vi "Configure Spectral (Other).vi"(0 "VISA resource name":refnum<visa-resource-name>, 1 "Frequency Span (100kHz)":dbl=100000.0, 2 "Resolution BW (400Hz)":dbl=400000.0, 3 "Gate Position (0s)":dbl, 5 "Channel (4:Math1)":u16(ring)=4 items=["Math 1"=4, "Math 2"=5, "Math 3"=6, "Math 4"=7], 11 "error in (no error)":errorcluster, 14 "Window Type (0:Rectangular)":u16(ring) items=["Rectangular", "Hamming", "Hanning", "KaiserBessel", "Black-Harris", "Flattop2", "Gaussian", "TekExp"]) -> (4 "VISA resource name out":refnum<visa-resource-name>, 15 "error out":errorcluster)   [LabVIEW 2011, in "Tektronix 7000 Series.lvlib"]
doc: "Configures the spectral real and imaginary operation methods for the specified math waveform."
uses:
  Tektronix 7000 Series.lvlib
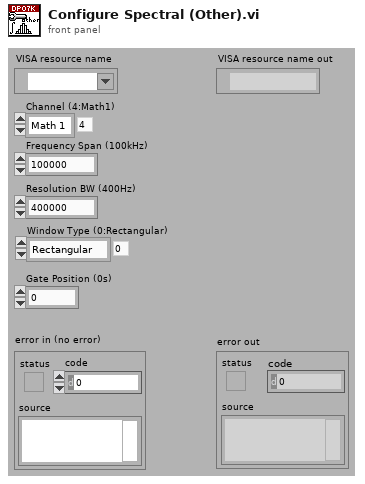
[diagram p1: front panel]
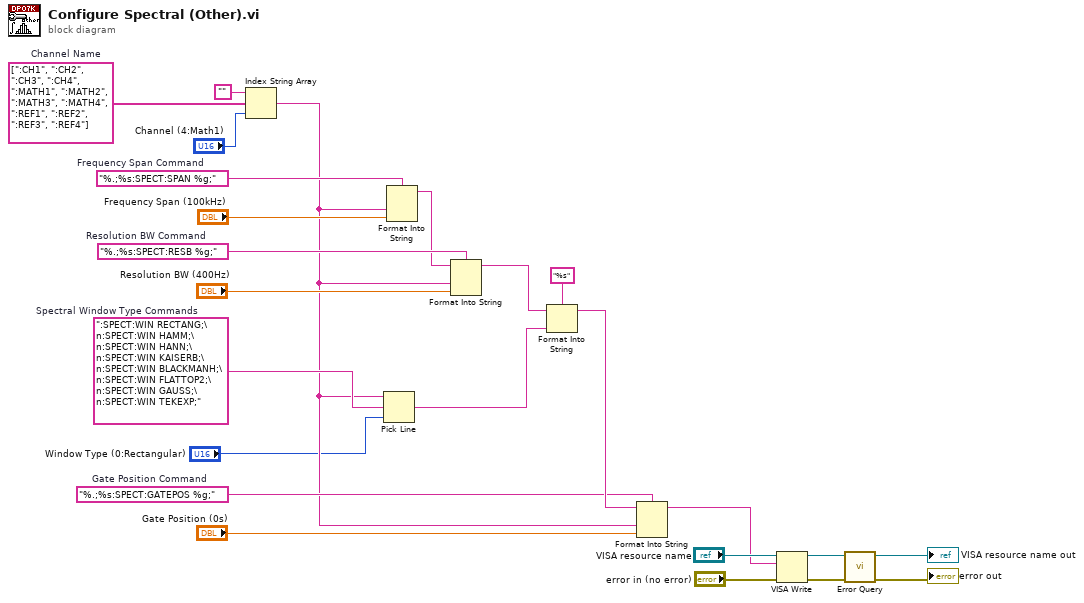
[diagram p0: block diagram]
diagram:
  w10 = "%.;%s:SPECT:GATEPOS %g;"  # Gate Position Command
  w18 = ":SPECT:WIN RECTANG;\n:SPECT:WIN HAMM;\n:SPECT:WIN HANN;\n:SPECT:WIN KAISERB;\n:SPECT:WIN BLACKMANH;\n:SPECT:WIN FLATTOP2;\n:SPECT:WIN GAUSS;\n:SPECT:WIN TEKEXP;"  # Spectral Window Type Commands
  w17 = "%.;%s:SPECT:RESB %g;"  # Resolution BW Command
  w15 = "%.;%s:SPECT:SPAN %g;"  # Frequency Span Command
  w24 = string[] [":CH1", ":CH2", ":CH3", ":CH4", ":MATH1", ":MATH2", ":MATH3", ":MATH4", ":REF1", ":REF2", ":REF3", ":REF4"]  # Channel Name
  n1 = Index String Array(1:"Channel (4:Math1)", 2:w24, 3:"") -> (0:w9:string)
  n2 = Pick Line(string ("")=w9, multi-line string=w18, line index="Window Type (0:Rectangular)") -> (output string=w21:string)
  n3 = Format Into String(format string=w15, w9, "Frequency Span (100kHz)") -> (resulting string=w16:string)  [unwired: 2 in, 1 out]
  n4 = Format Into String(format string=w17, initial string=w16, w9, "Resolution BW (400Hz)") -> (resulting string=w19:string)  [unwired: 1 in, 1 out]
  n5 = Format Into String(format string="%s", initial string=w19, w21) -> (resulting string=w12:string)  [unwired: 1 in, 1 out]
  n6 = Format Into String(format string=w10, initial string=w12, w9, "Gate Position (0s)") -> (resulting string=w2:string)  [unwired: 1 in, 1 out]
  n7 = VISA Write(VISA resource name="VISA resource name", write buffer=w2, error in (no error)="error in (no error)") -> (VISA resource name out=w8:refnum<visa-resource-name>, error out=w7:errorcluster)  [unwired: 1 out]
  n8 = call "Error Query.vi"("error in (no error)"=w7, "VISA resource name"=w8) -> ("error out"=→"error out":errorcluster, "VISA resource name out"=→"VISA resource name out":refnum<visa-resource-name>)  [unwired: 6 in, 2 out]
